vi "Process.vi"(8 "error in (no error)":errorcluster, 10 "Pound in":refnum<class "Pound.lvclass">, 11 "Qbus in":refnum<class "Qbus.lvclass">) -> (0 "error out":errorcluster)   [LabVIEW 2017, in "EmsaAcquisition.lvlib"]
uses:
  <vilib>/addons/InsightCM/Devices/Shared/Emsa/EmsaAcquisition/EmsaAcquisition.lvlib
  <vilib>/addons/Qbus/Qbus.lvclass
  <vilib>/NI/Software Watchdog/Pound/Pound.lvclass
  <vilib>/addons/InsightCM/Devices/Shared/Emsa/EmsaAcquisition/controls/config.ctl
  <vilib>/addons/InsightCM/Devices/Shared/Emsa/EmsaAcquisition/controls/group.ctl
  <vilib>/addons/InsightCM/Devices/Shared/Emsa/Emsa9770API/9770 API.lvclass
  <vilib>/addons/InsightCM/Devices/Shared/Emsa/EmsaAcquisition/controls/acqConfig.ctl
  <vilib>/addons/TraceLogger/TraceLogger.lvlib
  <vilib>/NI/Software Watchdog/Watchdog/Watchdog.lvclass
  <vilib>/addons/InsightCM/Devices/Shared/Common/FpgaBitfileManager/FpgaBitfileManager.lvlib
  <vilib>/addons/InsightCM/Devices/Shared/Emsa/EmsaDataEventCreator/EmsaDataEventCreator.lvlib
  <vilib>/addons/InsightCM/Devices/Shared/Emsa/EmsaAudio/EmsaAudio.lvlib
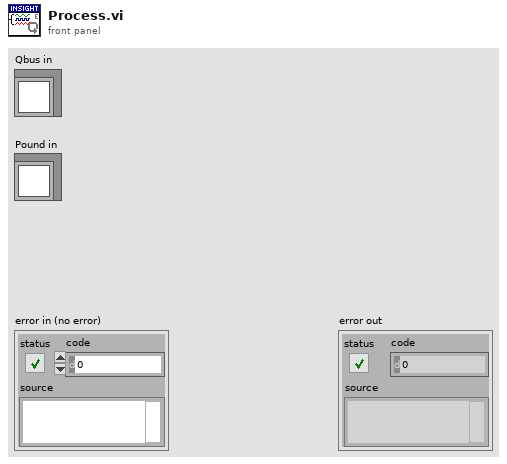
[diagram p1: front panel]
types:
  T1 = typedef "EmsaAcquisition.lvlib/config.ctl" = cluster{"FPGA reference":refnum<k20>, "Groups":T2[], "Acq Config":T3}
  T2 = typedef "EmsaAcquisition.lvlib/group.ctl" = cluster{"group name":string, "channels":refnum<class "9770 API.lvclass">[]}
  T3 = typedef "EmsaAcquisition.lvlib/acqConfig.ctl" = cluster{"channel":refnum<class "9770 API.lvclass">, "active":bool, "audio":bool, "total duration (samples)":i32, "duration (samples)":i32, "block size":i32, "bandwidth":dbl, "center frequency":dbl}
  T4 = typedef "EmsaDataEventCreator.lvlib/RegisterSweepRoutedMessage.ctl" = cluster{"Group":string, "Sweeps":T5[]}
  T5 = typedef "EmsaDataEventCreator.lvlib/Registry_Sweep.ctl" = cluster{"Name":string, "DataSetType":T6, "Properties":T7[]}
  T6 = typedef "DataEvent.lvlib/DataSetType.ctl" = enum16{"Waveform", "SpeedProfile", "ThermalImage", "EmsaSweep"}
  T7 = typedef "KeyValuePair.ctl" = cluster{"Key":string, "Value":string}
  T8 = typedef "EmsaAcquisition.lvlib/StartOnDemandAcquisitionRoutedMessage.ctl" = cluster{"Channel Name":string, "Audio":bool, "Center Frequency":dbl, "Bandwidth":dbl, "Duration":dbl, "Reference Level":dbl}
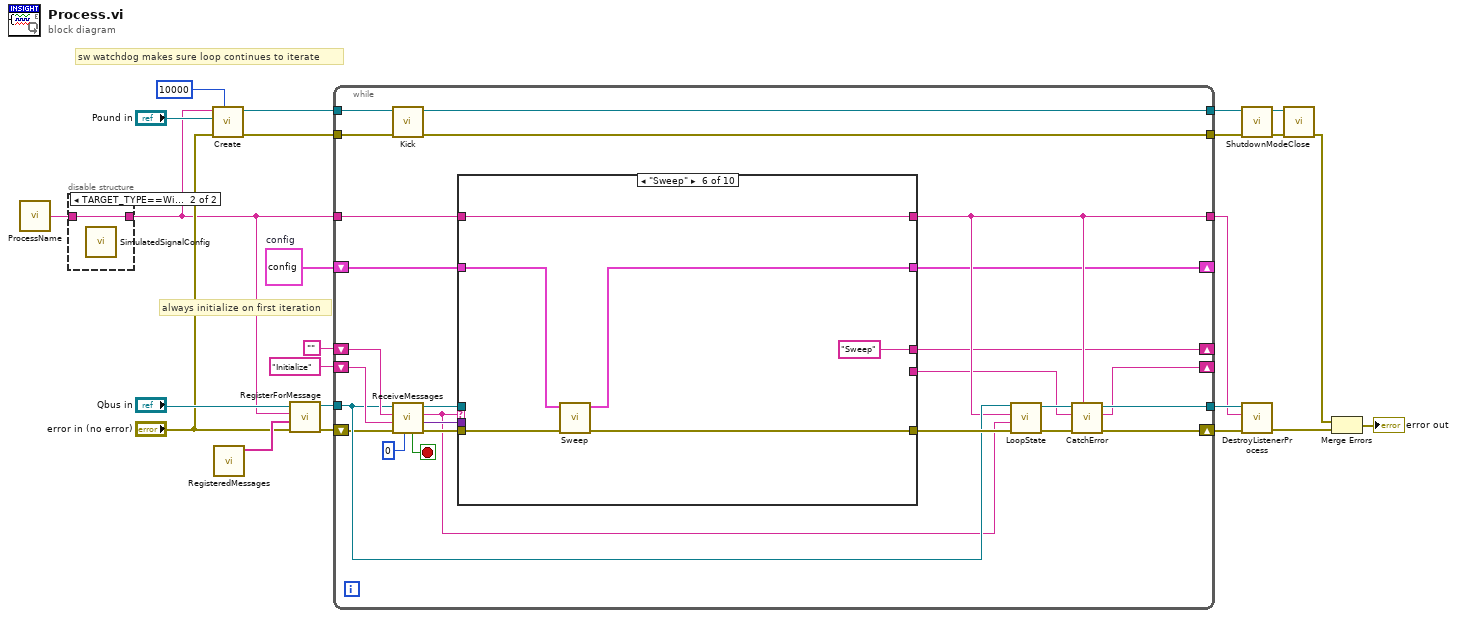
[diagram p0: block diagram]
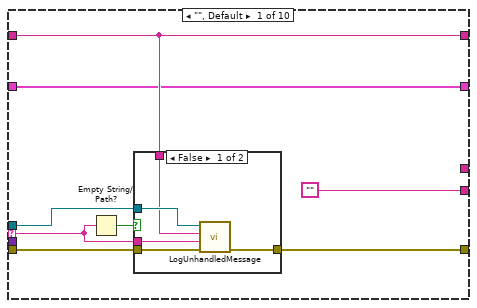
[diagram p3: hidden frame]
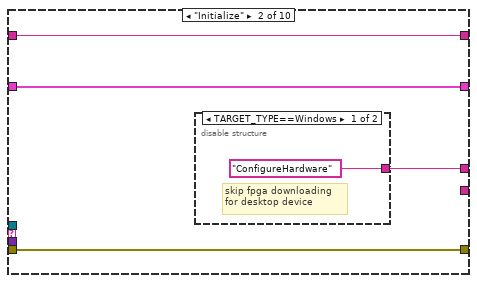
[diagram p5: hidden frame]
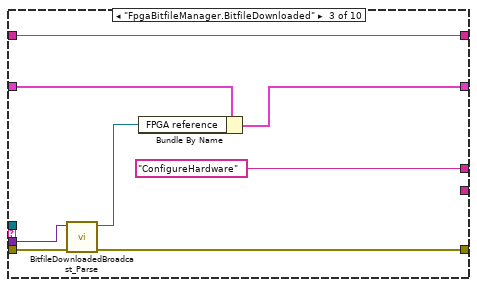
[diagram p7: hidden frame]
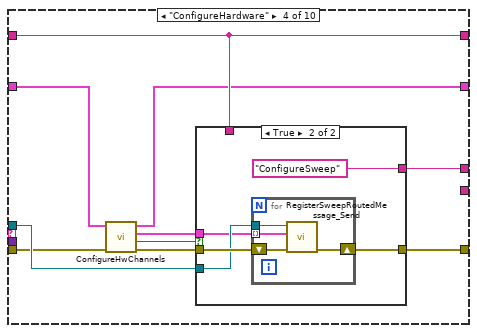
[diagram p8: hidden frame]
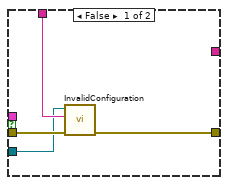
[diagram p9: hidden frame]
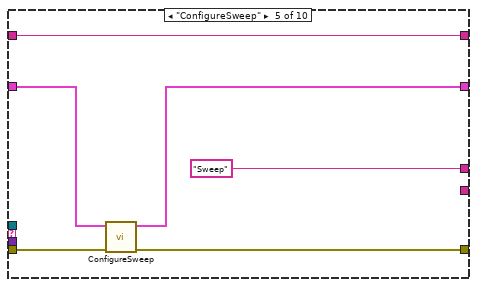
[diagram p10: hidden frame]
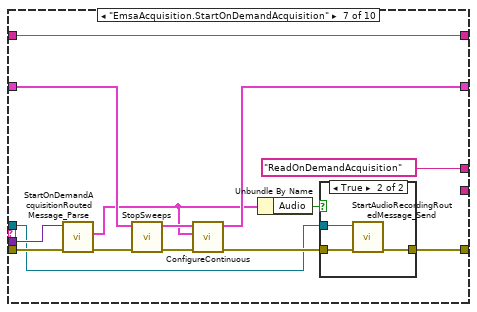
[diagram p11: hidden frame]
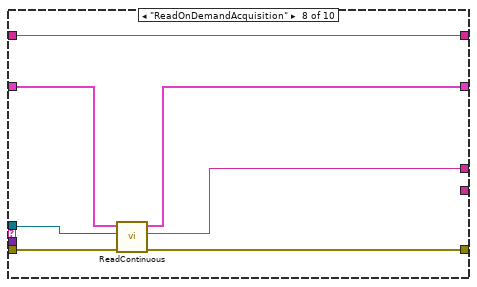
[diagram p13: hidden frame]
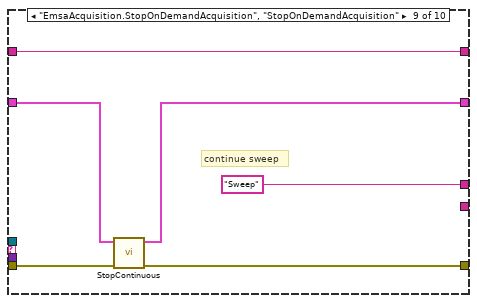
[diagram p14: hidden frame]
diagram:
  w3 = T1 {"FPGA reference"=refnum, "Groups"=[], "Acq Config"={"channel"=refnum, "active"=FALSE, "audio"=FALSE, "total duration (samples)"=0, "duration (samples)"=0, "block size"=0, "bandwidth"=0.0, "center frequency"=0.0}}  # config
  # "always initialize on first iteration"
  # "sw watchdog makes sure loop continues to iterate"
  n1 = call <vilib>:"ProcessName.vi"() -> ("process name"=w1:string)  [unwired: 5 in]
  n2 = disable-structure shown="TARGET_TYPE==Windows" {
    disable-tunnel: [w25 w26] -> w2
    disable-tunnel: w1 -> [w25 w26]
    frame condition #0 {
    }
    frame condition #1 (active) {
      n3 = call <vilib>:"SimulatedSignalConfig.vi"() -> ()  [unwired: 12 in]
    }
  }
  n4 = call <vilib>:"Create.vi"("Execution Timeout (ms)"=u32 10000, "error in (no error)"="error in (no error)", "Pound"="Pound in", "Name"=w2) -> ("error out"=w9:errorcluster, "Watchdog"=w15:refnum<data-value>)  [unwired: 6 in]
  n5 = call <vilib>:"RegisteredMessages.vi"() -> ("registered messages"=w16:string[])  [unwired: 11 in]
  n6 = call <vilib>:"RegisterForMessage.vi"("error in (no error)"="error in (no error)", "message names"=w16, "process name"=w2, "Qbus in"="Qbus in") -> ("error in (no error)"=w23:errorcluster, "Qbus out"=w22:refnum<class "Qbus.lvclass">)  [unwired: 6 in]
  n7 = while {
    shift-right: [w29] -> _
    shift-left: "" -> [w51]
    tunnel: w22 -> [w42]
    tunnel: w2 -> [w32]
    tunnel: [w45] -> w20
    tunnel: [w31] -> w19
    shift-right: [w44] -> _
    shift-left: "Initialize" -> [w47]
    tunnel: w15 -> [w41]
    tunnel: [w40] -> w11
    tunnel: w9 -> [w39]
    tunnel: [w37] -> w8
    shift-right: [w46] -> w21
    shift-left: w23 -> [w38]
    shift-right: [w27] -> _
    shift-left: w3 -> [w28]
    stop <- w52 stop-if-true
    n8 = call <vilib>:"Kick.vi"("error in (no error)"=w39, "Watchdog"=w41) -> ("error out"=w37:errorcluster, "Watchdog"=w40:refnum<data-value>)  [unwired: 8 in]
    n9 = call <vilib>:"ReceiveMessages.vi"("Timeout(1000)"=0 ("milliseconds to wait"), "error in (no error)"=w38, "priority action"=w47, "default action"=w51, "Qbus in"=w42) -> ("error out"=w50:errorcluster, "message value"=w48:variant, "action"=w36:string, "Qbus out"=w49:refnum<class "Qbus.lvclass">, "exit"=w52:bool)  [unwired: 2 in]
    n10 = case shown="\"Sweep\"" w36 {
      selector: w36 -> [w58 _ _ _ _ _ _ _ _ _]
      tunnel: w50 -> [w60 w67 w78 w82 w107 w114 w127 w138 w144 w148]
      tunnel: w49 -> [w56 _ _ w86 _ _ w115 w135 _ _]
      tunnel: [w59 w67 w73 w87 w106 w113 w119 w137 w143 w148] -> w43
      tunnel: w48 -> [_ _ w77 _ _ _ w116 _ _ _]
      tunnel: [w55 w70 w79 w85 w108 w111 w128 w139 w145 w147] -> w31
      tunnel: w32 -> [w55 w70 w79 w85 w108 w111 w128 w139 w145 w147]
      tunnel: ["" _ _ _ _ _ _ _ _ _] -> w30
      tunnel: [_ w69 "ConfigureHardware" w84 "Sweep" "Sweep" "ReadOnDemandAcquisition" w133 "Sweep" _] -> w29
      tunnel: w28 -> [w54 w68 w76 w81 w104 w109 w125 w136 w141 w146]
      tunnel: [w54 w68 w74 w80 w103 w110 w121 w134 w140 w146] -> w27
      frame "", Default {
        n11 = Empty String/Path?(string/path=w58) -> (empty?=w57:bool)
        n12 = case shown="False" w57 {
          tunnel: [w64 w66] -> w59
          tunnel: w60 -> [w65 w66]
          tunnel: w58 -> [w62 _]
          tunnel: w56 -> [w63 _]
          tunnel: w55 -> [w61 _]
          frame False {
            n13 = call <vilib>:"LogUnhandledMessage.vi"("error in (no error)"=w65, "message"=w62, "process"=w61, "Qbus in"=w63) -> ("error out"=w64:errorcluster)  [unwired: 7 in]
          }
          frame True {
          }
        }
      }
      frame "Initialize" {
        n14 = disable-structure shown="TARGET_TYPE==Windows" {
          disable-tunnel: ["ConfigureHardware" _] -> w69
          frame condition #0 (active) {
            # "skip fpga downloading\nfor desktop device"
          }
          frame condition #1 {
          }
        }
      }
      frame "FpgaBitfileManager.BitfileDownloaded" {
        n15 = call <vilib>:"BitfileDownloadedBroadcast_Parse.vi"("error in (no error)"=w78, "data"=w77) -> ("error out"=w73:errorcluster, "FPGA reference"=w75:refnum<k20>)  [unwired: 8 in]
        n16 = Bundle By Name(cluster=w76, "FPGA reference"=w75) -> (w74:T1)
      }
      frame "ConfigureHardware" {
        n17 = call <vilib>:"ConfigureHwChannels.vi"("error in (no error)"=w82, "config"=w81) -> ("error out"=w89:errorcluster, "valid"=w88:bool, "register sweeps"=w83:T4[], "config out"=w80:T1)  [unwired: 6 in]
        n18 = case shown="True" w88 {
          tunnel: [w93 w96] -> w87
          tunnel: w89 -> [w91 w97]
          tunnel: w85 -> [w92 _]
          tunnel: w86 -> [w90 w95]
          tunnel: [_ "ConfigureSweep"] -> w84
          tunnel: w83 -> [_ w94]
          frame False {
            n19 = call <vilib>:"InvalidConfiguration.vi"("error in (no error)"=w91, "description"=w92, "Qbus in"=w90) -> ("error out"=w93:errorcluster)  [unwired: 7 in, 1 out]
          }
          frame True {
            n20 = for {
              shift-right: [w100] -> w96
              shift-left: w97 -> [w101]
              tunnel: w94 -> [w99] mode=indexing
              tunnel: w95 -> [w102]
              n21 = call <vilib>:"RegisterSweepRoutedMessage_Send.vi"("error in (no error)"=w101, "RegisterSweepRoutedMessage"=w99, "Qbus in"=w102) -> ("error out"=w100:errorcluster)  [unwired: 7 in, 1 out]
            }
          }
        }
      }
      frame "ConfigureSweep" {
        n22 = call <vilib>:"ConfigureSweep.vi"("error in (no error)"=w107, "config"=w104) -> ("error out"=w106:errorcluster, "config out"=w103:T1)  [unwired: 8 in]
      }
      frame "Sweep" {
        n23 = call <vilib>:"Sweep.vi"("error in (no error)"=w114, "config"=w109) -> ("error out"=w113:errorcluster, "config out"=w110:T1)  [unwired: 8 in]
      }
      frame "EmsaAcquisition.StartOnDemandAcquisition" {
        n24 = call <vilib>:"StartOnDemandAcquisitionRoutedMessage_Parse.vi"("error in (no error)"=w127, "message"=w116) -> ("error out"=w124:errorcluster, "on demand acq config"=w120:T8)  [unwired: 8 in]
        n25 = call <vilib>:"StopSweeps.vi"("error in (no error)"=w124, "config"=w125) -> ("error out"=w123:errorcluster, "config out"=w122:T1)  [unwired: 8 in]
        n26 = call <vilib>:"ConfigureContinuous.vi"("error in (no error)"=w123, "on demand acq config"=w120, "config"=w122) -> ("error out"=w118:errorcluster, "config out"=w121:T1)  [unwired: 7 in]
        n27 = Unbundle By Name(w120) -> ("Audio"=w117:bool)
        n28 = case shown="True" w117 {
          tunnel: [w129 w131] -> w119
          tunnel: w118 -> [w129 w132]
          tunnel: w115 -> [_ w130]
          frame False {
          }
          frame True {
            n29 = call <vilib>:"StartAudioRecordingRoutedMessage_Send.vi"("error in (no error)"=w132, "Qbus in"=w130) -> ("error out"=w131:errorcluster)  [unwired: 8 in, 1 out]
          }
        }
      }
      frame "ReadOnDemandAcquisition" {
        n30 = call <vilib>:"ReadContinuous.vi"("error in (no error)"=w138, "Qbus in"=w135, "config"=w136) -> ("error out"=w137:errorcluster, "next action"=w133:string, "cofig out"=w134:T1)  [unwired: 6 in]
      }
      frame "EmsaAcquisition.StopOnDemandAcquisition", "StopOnDemandAcquisition" {
        # "continue sweep"
        n31 = call <vilib>:"StopContinuous.vi"("error in (no error)"=w144, "config"=w141) -> ("error out"=w143:errorcluster, "config out"=w140:T1)  [unwired: 8 in]
      }
      frame "Exit" {
      }
    }
    n32 = call <vilib>:"LoopState.vi"("error in (no error)"=w43, "loop action"=w36, "process name"=w31, "Qbus in"=w42) -> ("error out"=w34:errorcluster, "Qbus out"=w33:refnum<class "Qbus.lvclass">)  [unwired: 6 in]
    n33 = call <vilib>:"CatchError.vi"("source"=w31, "error in (no error)"=w34, "next action in"=w30, "Qbus in"=w33) -> ("error out"=w46:errorcluster, "next action out"=w44:string, "Qbus out"=w45:refnum<class "Qbus.lvclass">)  [unwired: 5 in]
  }
  n34 = call <vilib>:"ShutdownMode.vi"("error in (no error)"=w8, "Watchdog"=w11) -> ("error out"=w10:errorcluster, "Watchdog"=w12:refnum<data-value>)  [unwired: 8 in]
  n35 = call <vilib>:"DestroyListenerProcess.vi"("error in (no error)"=w21, "process name"=w19, "Qbus in"=w20) -> ("error in (no error)"=w7:errorcluster)  [unwired: 7 in, 1 out]
  n36 = call <vilib>:"Close.vi"("error in (no error)"=w10, "Watchdog"=w12) -> ("error out"=w6:errorcluster)  [unwired: 9 in]
  n37 = Merge Errors(w6, w7) -> (→"error out":errorcluster)
